vi "Find Packed Library.vi"(8 "error in (no error)":errorcluster, 10 "packed library name":string, 11 "Component Loader in":refnum<class "Component Loader.lvclass">) -> (0 "error out":errorcluster, 2 "packed library path":path, 3 "Component Loader out":refnum<class "Component Loader.lvclass">)   [LabVIEW 2017, in "Data Sharing Framework Engine.lvlib" / "Component Loader.lvclass"]
uses:
  Component Loader.lvclass
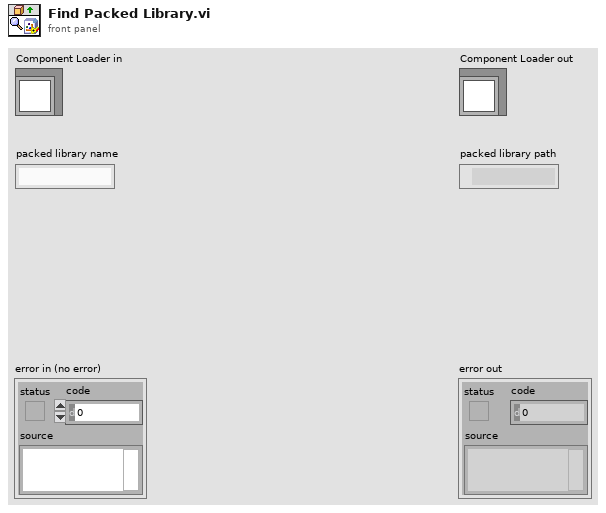
[diagram p1: front panel]
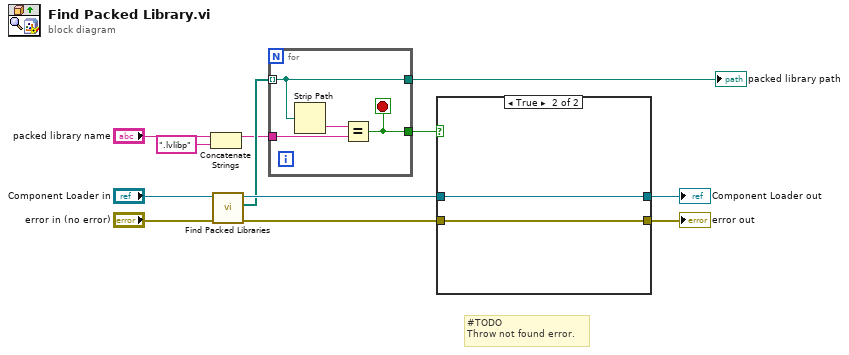
[diagram p0: block diagram]
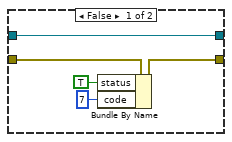
[diagram p2: hidden frame]
diagram:
  # "#TODO\nThrow not found error."
  n1 = Concatenate Strings("packed library name", ".lvlibp" ("string")) -> (w1:string)
  n2 = call "Find Packed Libraries.vi"("error in (no error)"="error in (no error)", "Component Loader in"="Component Loader in") -> ("error out"=w7:errorcluster, "packed library paths"=w4:path[], "Component Loader out"=w8:refnum<class "Component Loader.lvclass">)  [unwired: 7 in]
  n3 = for {
    tunnel: w4 -> [w14] mode=indexing
    tunnel: w1 -> [w15]
    tunnel: [w14] -> w10
    tunnel: [w13] -> w9
    stop <- w13 stop-if-true
    n4 = Strip Path(path=w14) -> (name=w16:string)  [unwired: 1 out]
    n5 = Equal?(x=w16, y=w15) -> (x = y?=w13:bool)
  }
  "packed library path" <- w10
  n6 = case shown="True" w9 {
    tunnel: w8 -> [w21 w23]
    tunnel: w7 -> [w20 w22]
    tunnel: [w21 w23] -> w6
    tunnel: [w19 w22] -> w5
    frame False {
      n7 = Bundle By Name(cluster=w20, "status"=TRUE, "code"=7) -> (w19:errorcluster)
    }
    frame True {
    }
  }
  "error out" <- w5
  "Component Loader out" <- w6
